vi "BS1200-v2 Discovery Parser.vi"(10 "IP Address":string, 11 "Discovery String":string) -> (3 "Devices":T1[](array[typedef]))   [LabVIEW 2021, in "BS120x Driver.lvlib"]
uses:
  BS120x Driver.lvlib
  New BS120x Device/DiscoveredDevice.ctl
  TypeDefs/UnitType.ctl
  TypeDefs/Protocol.ctl
  BS120x.lvclass
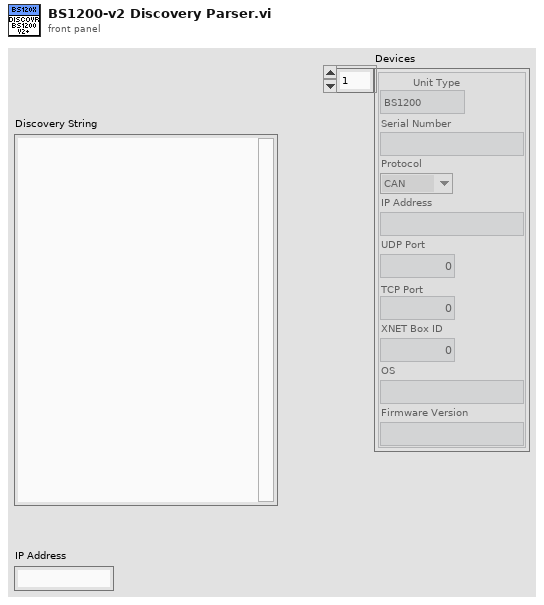
[diagram p1: front panel]
types:
  T1 = typedef "BS120x Driver.lvlib/DiscoveredDevice.ctl" = cluster{"Unit Type":T2, "Serial Number":string, "Protocol":T3, "IP Address":string, "UDP Port":u16, "TCP Port":u16, "XNET Box ID":u8, "OS":string, "Firmware Version":string}
  T2 = typedef "BS120x Driver.lvlib/BS120x.lvclass/UnitType.ctl" = enum16{"BS1200", "BS1201"}
  T3 = typedef "BS120x Driver.lvlib/BS120x.lvclass/Protocol.ctl" = enum16{"CAN", "Ethernet"}
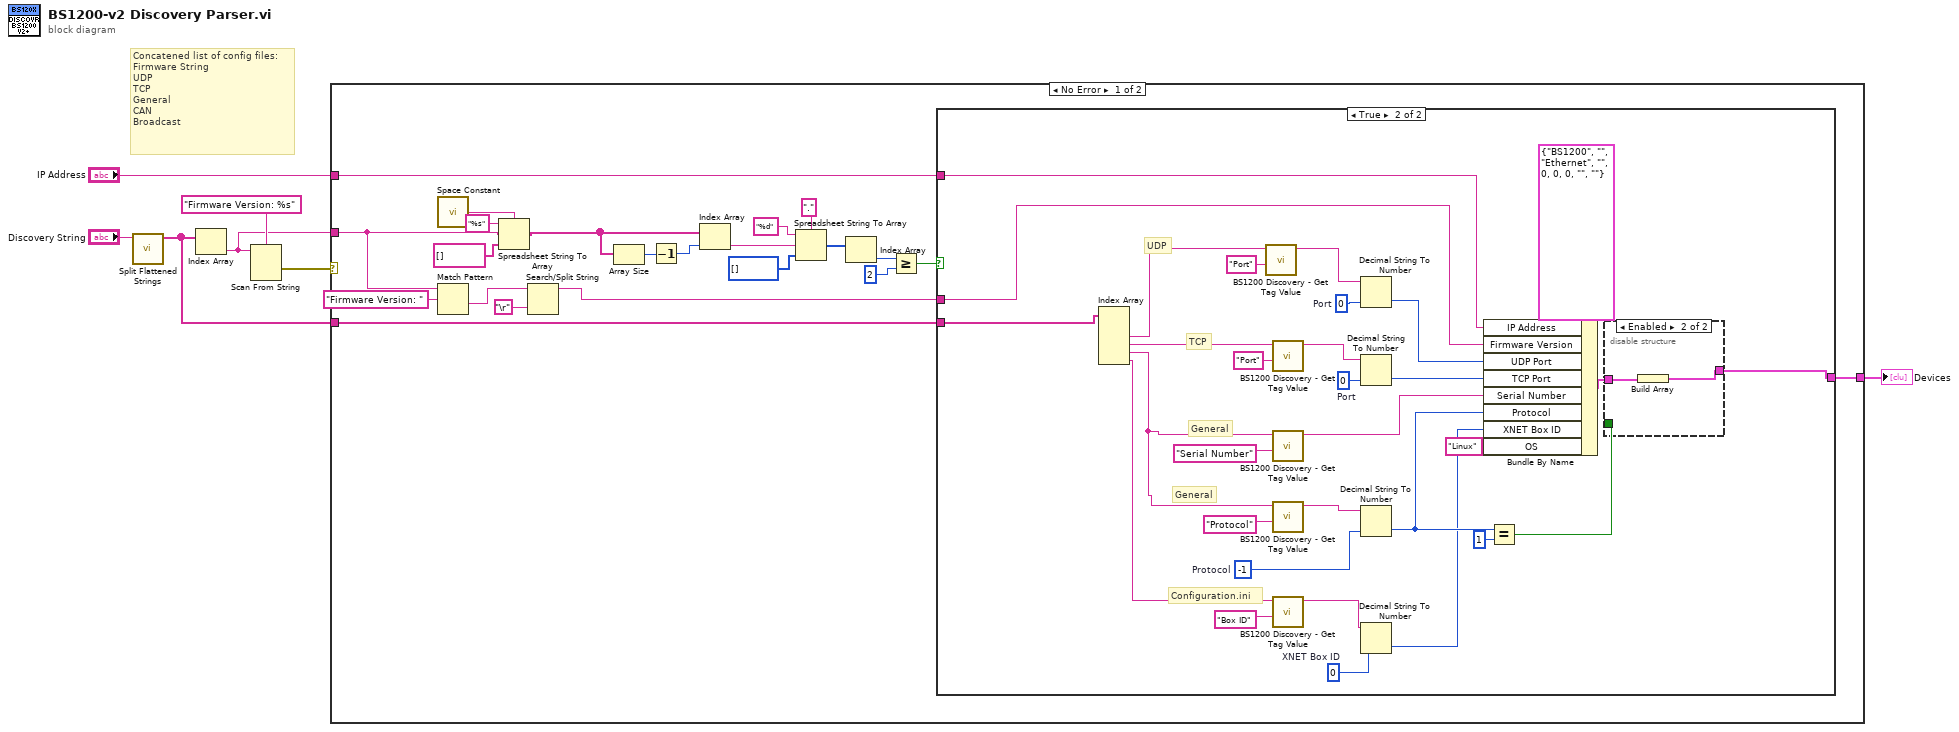
[diagram p0: block diagram]
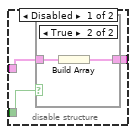
[diagram p3: hidden frame]
diagram:
  # "Concatened list of config files:\nFirmware String\nUDP\nTCP\nGeneral\nCAN\nBroadcast"
  n1 = call "Split Flattened Strings.vi"("Flattened Strings"="Discovery String") -> ("Strings"=w5:string[])  [unwired: 10 in]
  n2 = Index Array(array=w5) -> (element=w2:string)  [unwired: 1 in]
  n3 = Scan From String(format string="Firmware Version: %s", input string=w2) -> (error out=w4:errorcluster)  [unwired: 4 in, 2 out]
  n4 = case shown="No Error" w4 {
    tunnel: [w29 _] -> w6
    tunnel: w5 -> [w28 _]
    tunnel: w2 -> [w12 _]
    tunnel: "IP Address" -> [w17 _]
    frame No Error {
      n5 = call <vilib>:"Space Constant.vi"() -> ("String"=w16:string)
      n6 = Match Pattern(string=w12, regular expression="Firmware Version: ") -> (after substring=w10:string)  [unwired: 1 in, 3 out]
      n7 = Spreadsheet String To Array(delimiter (Tab)=w16, format string="%s", spreadsheet string=w12, array type (2D Dbl)=string[] []) -> (array=w13:string[])
      n8 = Search/Split String(string=w10, search string/char (-)="\r") -> (substring before match=w8:string)  [unwired: 1 in, 2 out]
      n9 = Array Size(array=w13) -> (size(s)=w27:i32)
      n10 = Decrement(x=w27) -> (x-1=w26:i32)
      n11 = Index Array(array=w13, index=w26) -> (element=w25:string)
      n12 = Spreadsheet String To Array(delimiter (Tab)=".", format string="%d", spreadsheet string=w25, array type (2D Dbl)=i32[] []) -> (array=w21:i32[])
      n13 = Index Array(array=w21) -> (element=w20:i32)  [unwired: 1 in]
      n14 = Greater Or Equal?(x=w20, y=2) -> (x >= y?=w18:bool)
      n15 = case shown="True" w18 {
        tunnel: w28 -> [_ w34]
        tunnel: [_ w32] -> w29
        tunnel: w17 -> [_ w33]
        tunnel: w8 -> [_ w30]
        frame False {
        }
        frame True {
          w36 = u8 0  # XNET Box ID
          w57 = u16 0  # Port
          w58 = -1  # Protocol
          w60 = u16 0  # Port
          # "Configuration.ini"
          # "General"
          # "General"
          # "TCP"
          # "UDP"
          n16 = Index Array(array=w34) -> (element #2=w51:string, element #3=w47:string, element #4=w45:string, element #5=w40:string)  [unwired: 5 in, 1 out]
          n17 = call "BS1200 Discovery - Get Tag Value.vi"("Name"="Port", "Input String"=w51) -> ("Value"=w49:string)  [unwired: 9 in]
          n18 = call "BS1200 Discovery - Get Tag Value.vi"("Name"="Port", "Input String"=w47) -> ("Value"=w46:string)  [unwired: 9 in]
          n19 = call "BS1200 Discovery - Get Tag Value.vi"("Name"="Serial Number" ("Initial Filter"), "Input String"=w45) -> ("Value"=w35:string)  [unwired: 9 in]
          n20 = call "BS1200 Discovery - Get Tag Value.vi"("Name"="Protocol" ("Initial Filter"), "Input String"=w45) -> ("Value"=w43:string)  [unwired: 9 in]
          n21 = call "BS1200 Discovery - Get Tag Value.vi"("Name"="Box ID" ("Initial Filter"), "Input String"=w40) -> ("Value"=w38:string)  [unwired: 9 in]
          n22 = Decimal String To Number(string=w49, default (0L)=w60) -> (number=w59:u16)  [unwired: 1 in, 1 out]
          n23 = Decimal String To Number(string=w46, default (0L)=w57) -> (number=w56:u16)  [unwired: 1 in, 1 out]
          n24 = Decimal String To Number(string=w43, default (0L)=w58) -> (number=w39:i32)  [unwired: 1 in, 1 out]
          n25 = Decimal String To Number(string=w38, default (0L)=w36) -> (number=w37:u8)  [unwired: 1 in, 1 out]
          n26 = Bundle By Name(cluster=T1 {"Unit Type"=enum."BS1200", "Serial Number"="", "Protocol"=enum."Ethernet", "IP Address"="", "UDP Port"=0, "TCP Port"=0, "XNET Box ID"=0, "OS"="", "Firmware Version"=""} ("Device"), "IP Address"=w33, "Firmware Version"=w30, "UDP Port"=w59, "TCP Port"=w56, "Serial Number"=w35, "Protocol"=w39, "XNET Box ID"=w37, "OS"="Linux" ("Comment")) -> (w53:T1)
          n27 = Equal?(x=w39, y=1) -> (x = y?=w52:bool)
          n28 = disable-structure shown="Enabled" {
            disable-tunnel: w53 -> [w63 w67]
            disable-tunnel: w52 -> [w62 _]
            disable-tunnel: [w61 w66] -> w32
            frame Disabled {
              n29 = case shown="True" w62 {
                tunnel: w63 -> [_ w65]
                tunnel: [_ w64] -> w61
                frame False {
                }
                frame True {
                  n30 = Build Array(w65) -> (w64:T1[])
                }
              }
            }
            frame Enabled {
              n31 = Build Array(w67) -> (w66:T1[])
            }
          }
        }
      }
    }
    frame Error {
    }
  }
  "Devices" <- w6
